vi "SetDyeStrings.vi"(8 "error in (no error)":errorcluster, 10 "Select Dye:":refnum<vi>, 11 "Settings in":refnum<class "Settings.lvclass">) -> (0 "error out":errorcluster, 1 "Excitation String":string, 2 "Emission Filter String":string, 3 "Settings out":refnum<class "Settings.lvclass">)   [LabVIEW 2010, in "Settings.lvclass"]
uses:
  Settings.lvclass
  Settings.lvclass/Settings.ctl
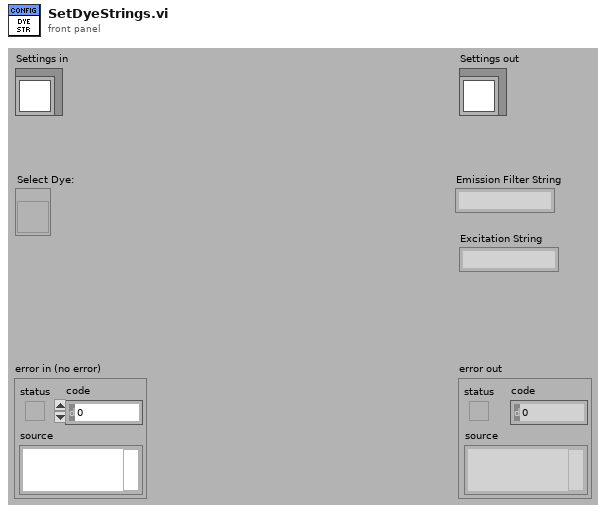
[diagram p1: front panel]
types:
  T1 = cluster{"Dye Name":string, "Pulse Sequence":cluster{"LED Name":string, "Pulse Length (s)":dbl, "Delay Before (s)":dbl, "Delay After (s)":dbl, "Trigger Camera":bool}[], "Emission Filter":i16, "Exposure (s)":dbl, "Yellow Select":bool, "# Pulses":i32}[]
  T2 = cluster{"Color":string, "Wavelength":i32, "Wheel Position":i32}[]
  T3 = cluster{"Dye Name":string, "Pulse Sequence":cluster{"LED Name":string, "Pulse Length (s)":dbl, "Delay Before (s)":dbl, "Delay After (s)":dbl, "Trigger Camera":bool}[], "Emission Filter":i16, "Exposure (s)":dbl, "Yellow Select":bool, "# Pulses":i32}
  T4 = cluster{"LED Name":string, "Pulse Length (s)":dbl, "Delay Before (s)":dbl, "Delay After (s)":dbl, "Trigger Camera":bool}[]
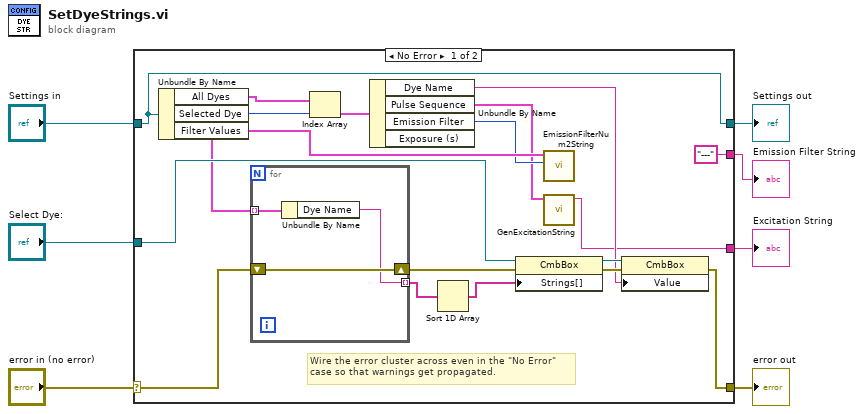
[diagram p0: block diagram]
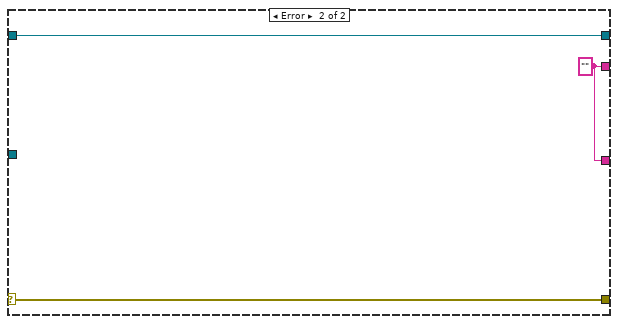
[diagram p2: hidden frame]
diagram:
  n1 = case shown="No Error" "error in (no error)" {
    selector: "error in (no error)" -> [w22 w31]
    tunnel: [w21 w31] -> w6
    tunnel: [w19 w30] -> w4
    tunnel: "Settings in" -> [w19 w30]
    tunnel: "Select Dye:" -> [w20 _]
    tunnel: ["---" ("Emission Filter String") w29] -> w2
    tunnel: [w11 w29] -> w1
    frame No Error {
      # "Wire the error cluster across even in the \"No Error\"\ncase so that warnings get propagated."
      n2 = Unbundle By Name(w19) -> ("All Dyes"=w18:T1, "Selected Dye"=w17:i32, "Filter Values"=w14:T2)
      n3 = for {
        tunnel: w18 -> [w28] mode=indexing
        shift-right: [w27] -> w23
        shift-left: w22 -> [w27]
        tunnel: [w26] -> w10 mode=indexing
        n4 = Unbundle By Name(w28) -> ("Dye Name"=w26:string)
      }
      n5 = Index Array(array=w18, index=w17) -> (element=w16:T3)
      n6 = Unbundle By Name(w16) -> ("Dye Name"=w15:string, "Pulse Sequence"=w12:T4, "Emission Filter"=w13:i16)  [unwired: 1 out]
      n7 = Sort 1D Array(array=w10) -> (sorted array=w9:string[])
      n8 = property on="Property Node" class="CmbBox"(reference=w20, error in=w23, "Strings[]"=w9) -> (reference out=w25:refnum<vi>, error out=w24:errorcluster)
      n9 = call "EmissionFilterNum2String.vi"("Emission Filter"=w13, "Filter Values"=w14) -> ()  [unwired: 9 in, 1 out]
      n10 = call "GenExcitationString.vi"("Pulse Sequence"=w12) -> ("Emission Filter String"=w11:string)  [unwired: 10 in]
      n11 = property on="Property Node" class="CmbBox"(reference=w25, error in=w24, "Value"=w15) -> (error out=w21:errorcluster)  [unwired: 1 out]
    }
    frame Error {
      w29 = "" ("Emission Filter String")
    }
  }
  "error out" <- w6
  "Settings out" <- w4
  "Emission Filter String" <- w2
  "Excitation String" <- w1
